vi "string front part.vi"(10 "字符串":string, 11 "偏移量(0)":i32) -> (3 "result string":string)   [LabVIEW 2019, in "SubVI.lvlib"]
uses:
  SubVI.lvlib
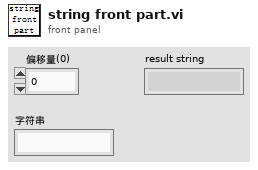
[diagram p1: front panel]
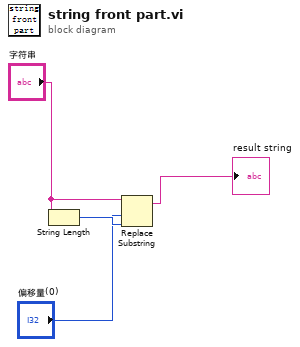
[diagram p0: block diagram]
diagram:
  n1 = String Length(string="字符串") -> (length=w2:i32)
  n2 = Replace Substring(2:w2, 3:"偏移量(0)", 5:"字符串") -> (1:→"result string":string)  [unwired: 1 in, 1 out]
